vi "Cursor Update.vi"(7 "XY Graph Ref":refnum<vi>, 8 "error in (no error)":errorcluster, 11 "Xinformation In":T1) -> (0 "error out":errorcluster, 3 "Xinformation Out":T1)   [LabVIEW 2015, in "Teaching View.lvlib" / "Teaching View XControl.xctl"]
doc: "Redraws the main waveform graph by using the cursor positions to update the waveform's scale range."
uses:
  Teaching View XControl.xctl
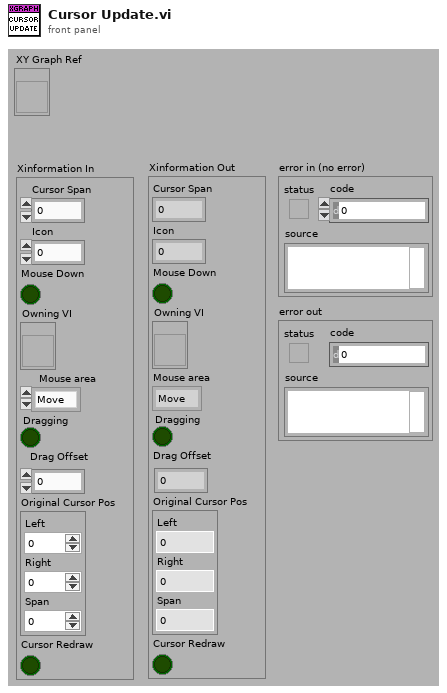
[diagram p1: front panel]
types:
  T1 = cluster{"Cursor Span":dbl, "Icon":u16, "Mouse Down":bool, "Owning VI":refnum<vi>, "Mouse area":enum16{"Move", "left cursor", "right cursor", "none"}, "Dragging":bool, "Drag Offset":dbl, "Original Cursor Pos":cluster{"Left":dbl, "Right":dbl, "Span":dbl}, "Cursor Redraw":bool}
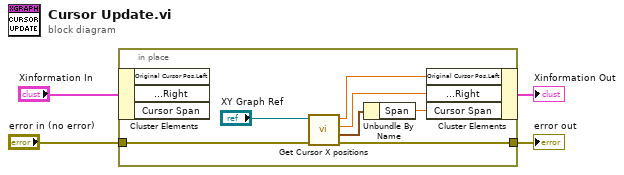
[diagram p0: block diagram]
diagram:
  n1 = in-place {
    in-place-border: "error in (no error)" -> [w9]
    in-place-border: [w8] -> w1
    n2 = in-place-cluster #1("Xinformation In") -> ()  [unwired: 3 out]
    n3 = call "Get Cursor X positions.vi"("error in"=w9, "XY Graph Ref"="XY Graph Ref") -> ("error out"=w8:errorcluster, "Cursors"=w11:cluster{"Left":dbl, "Right":dbl, "Span":dbl}, "Right"=w5:dbl, "Left"=w6:dbl)  [unwired: 6 in]
    n4 = Unbundle By Name(w11) -> ("Span"=w7:dbl)
    n5 = in-place-cluster #1("Original Cursor Pos.Left"=w6, "Original Cursor Pos.Right"=w5, "Cursor Span"=w7) -> (→"Xinformation Out":T1)
  }
  "error out" <- w1
